vi "main.vi"() -> ()   [LabVIEW 2020]
uses:
  states_enum_typedef.ctl
  <vilib>/Analysis/baseanly.llb/Mean (DBL).vi
  <vilib>/addons/control/pid/pid.llb/PID (DBL).vi
  <vilib>/Analysis/NI_AALBase.lvlib
  <vilib>/addons/control/pid/NI_PID_pid.lvlib
panel:
  in  "Exit":bool
  in  "Tab Control":enum32{"Control", "Notes", "Profile", "Setup"}(tab)
  out "Zone 3\n Chart":dbl(graph)
  out "Zone 2 Chart":dbl(graph)
  out "Zone 1 Chart":dbl(graph)
  in  "Zone 1 SP":dbl
  in  "Zone 2 SP":dbl
  in  "Zone 3 SP":dbl
  out "Zone 1 Duty Cycle":dbl(knob) scale=0.0..100.0
  out "Zone 2 Duty Cycle":dbl(knob) scale=0.0..100.0
  out "Zone 3 Duty Cycle":dbl(knob) scale=0.0..100.0
  out "Z1":bool
  out "Z2":bool
  out "Z3":bool
  in  "Notes":string
  out "Profile Chart":dbl(graph)
  in  "Reset":bool
  out "Control Loop Stopped":bool
  out "Main Loop":i32
  out "PWM Loop":i32
  in  "Zone 1 PID":T1={"proportional gain (Kc)"=1.0, "integral time (Ti, min)"=0.01, "derivative time (Td, min)"=0.0} {"derivative time (Td, min)" format="%.3f"; "integral time (Ti, min)" format="%.3f"; "proportional gain (Kc)" format="%.3f"}
  in  "Zone 2 PID":T1={"proportional gain (Kc)"=1.0, "integral time (Ti, min)"=0.01, "derivative time (Td, min)"=0.0} {"derivative time (Td, min)" format="%.3f"; "integral time (Ti, min)" format="%.3f"; "proportional gain (Kc)" format="%.3f"}
  in  "Zone 3 PID":T1={"proportional gain (Kc)"=1.0, "integral time (Ti, min)"=0.01, "derivative time (Td, min)"=0.0} {"derivative time (Td, min)" format="%.3f"; "integral time (Ti, min)" format="%.3f"; "proportional gain (Kc)" format="%.3f"}
  out "Errors":errorcluster
  out "PWM Errors":errorcluster
  out "Zone 3":dbl(slide) scale=15.0..350.0
  out "Zone 2":dbl(slide) scale=15.0..350.0
  out "Zone 1":dbl(slide) scale=15.0..350.0
  # "Reflow Oven Controller"
  # "DegC"
  # "DegC"
  # "DegC"
  # "Any notes you type here will be saved and is a handy pad for future reference"
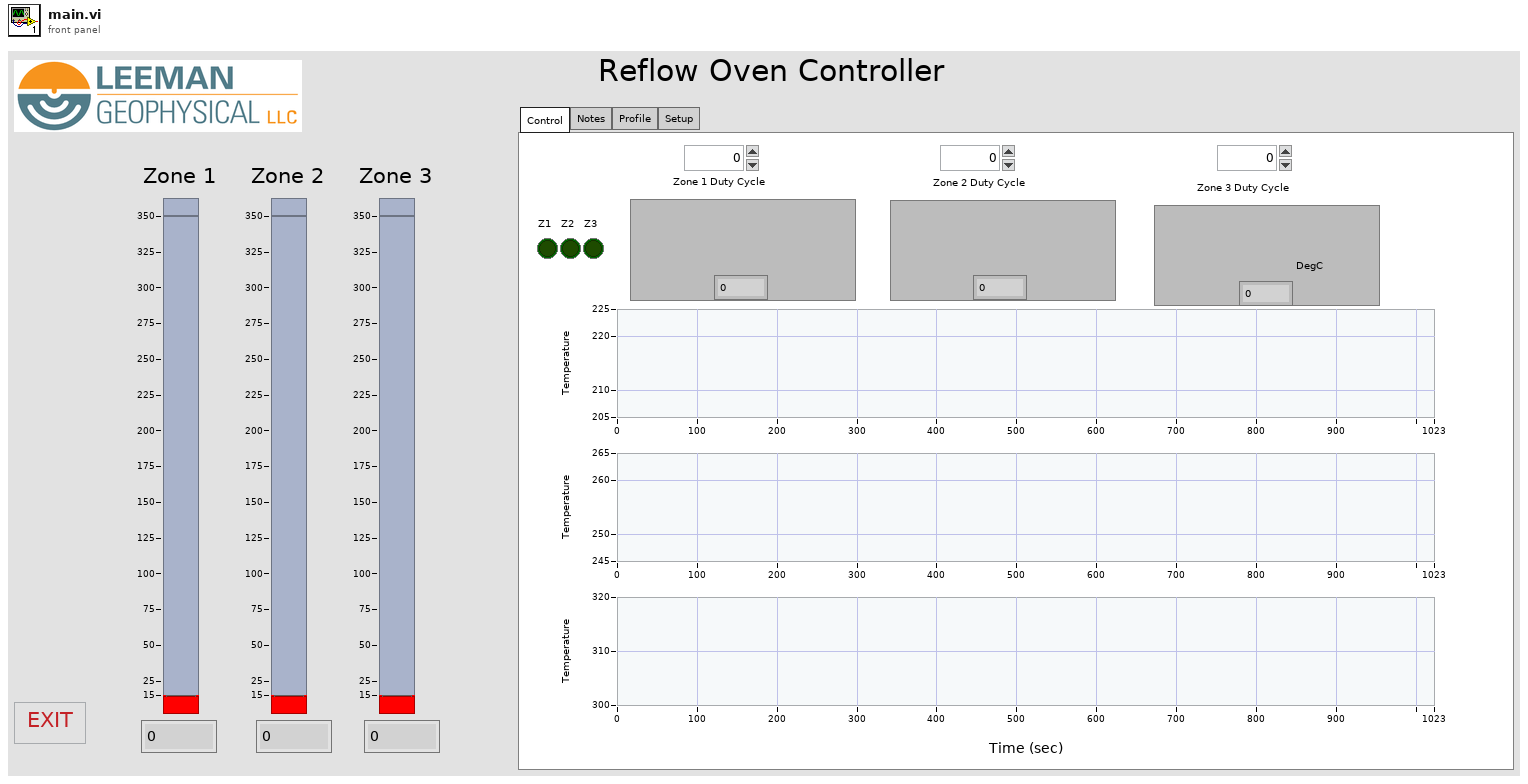
[diagram p1: front panel]
types:
  T1 = cluster{"proportional gain (Kc)":dbl, "integral time (Ti, min)":dbl, "derivative time (Td, min)":dbl}
  T2 = typedef "states_enum_typedef.ctl" = enum16{"Initilize", "Read", "Control 1", "Control 2", "Control 3", "Reset", "Wait", "Shutdown"}
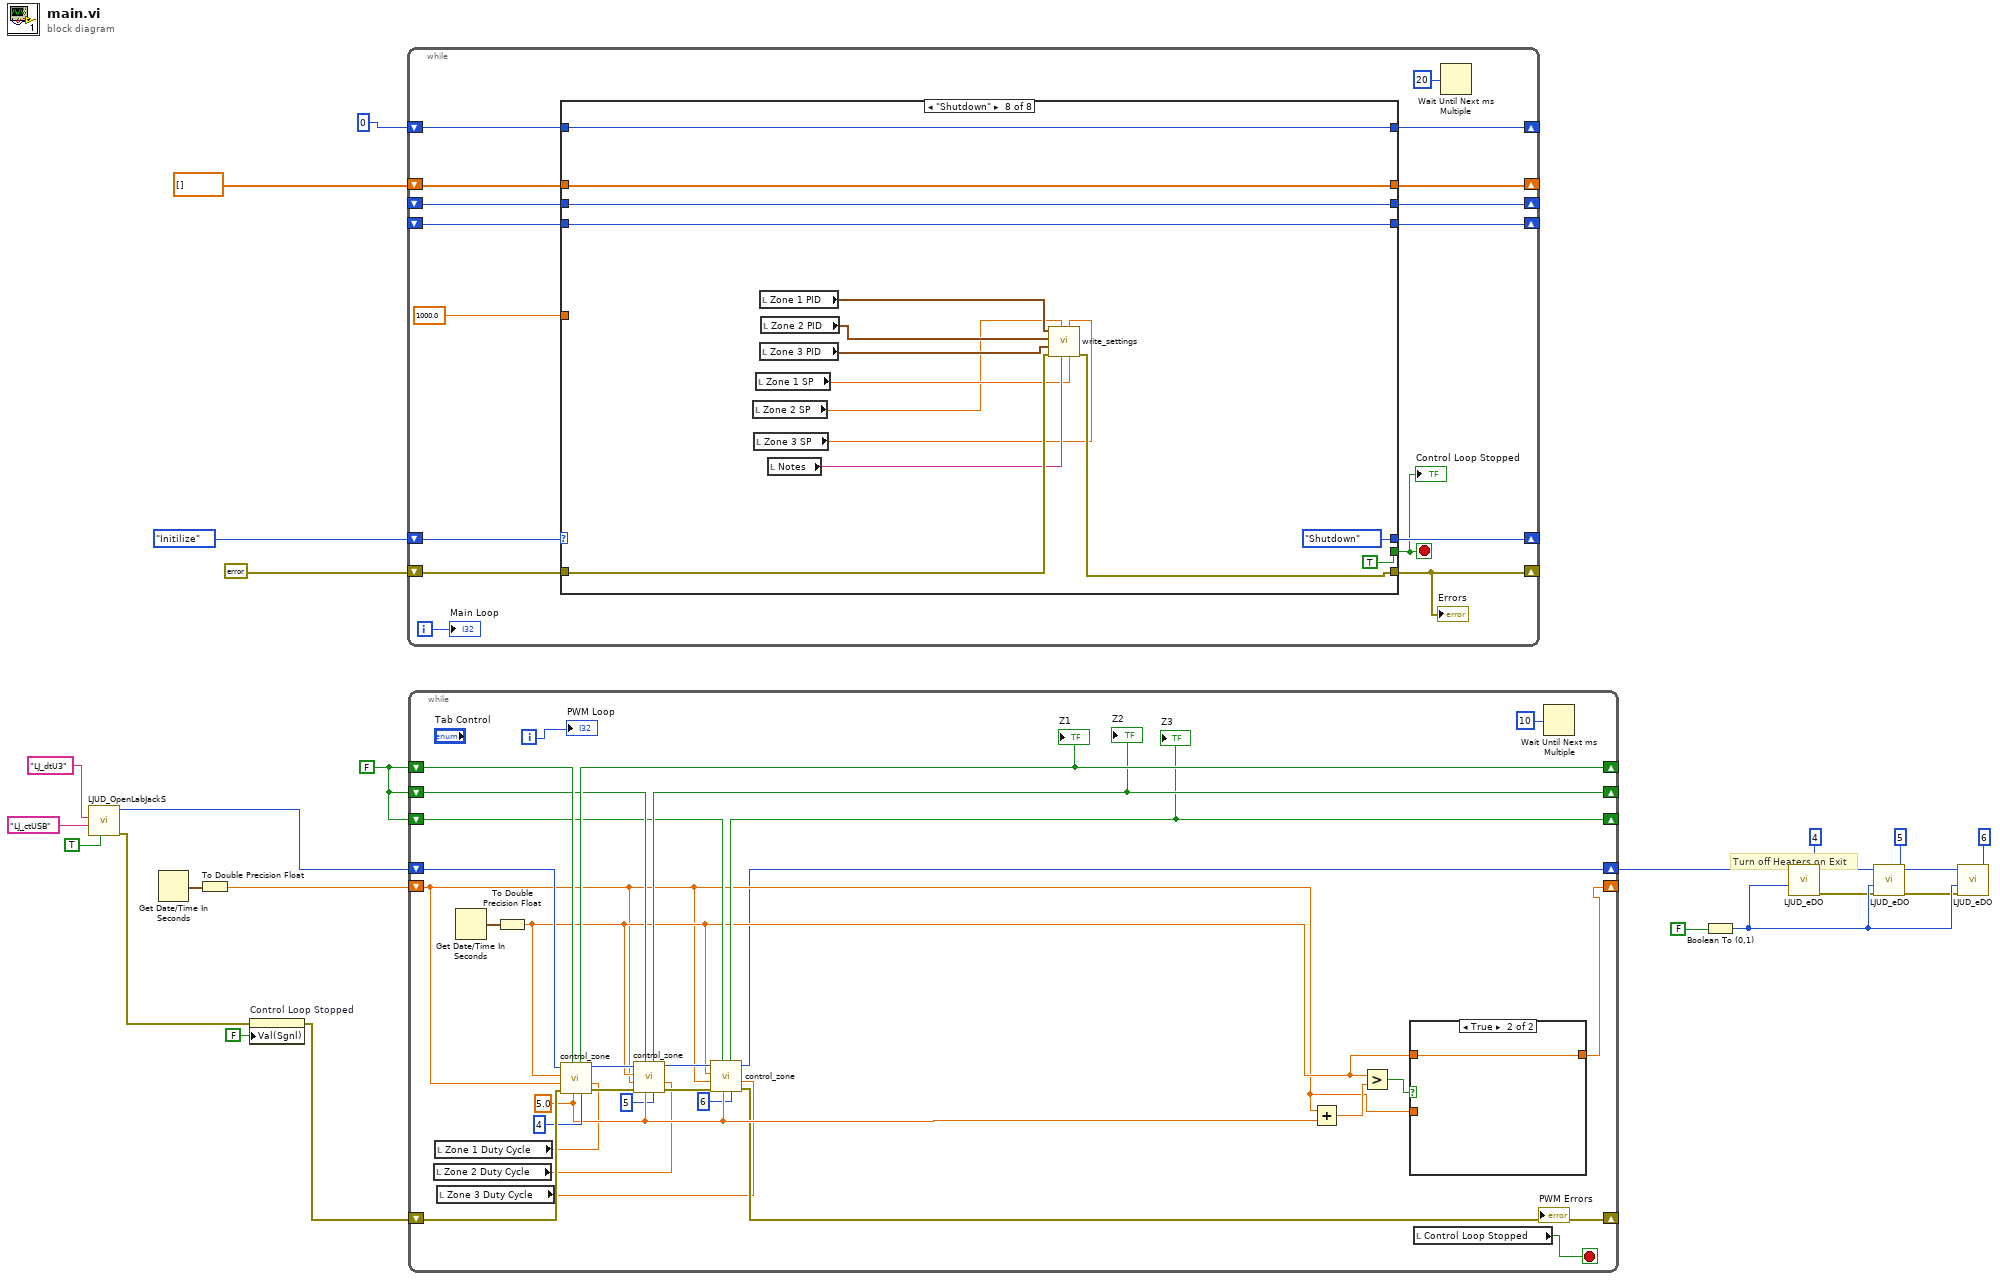
[diagram p0: block diagram]
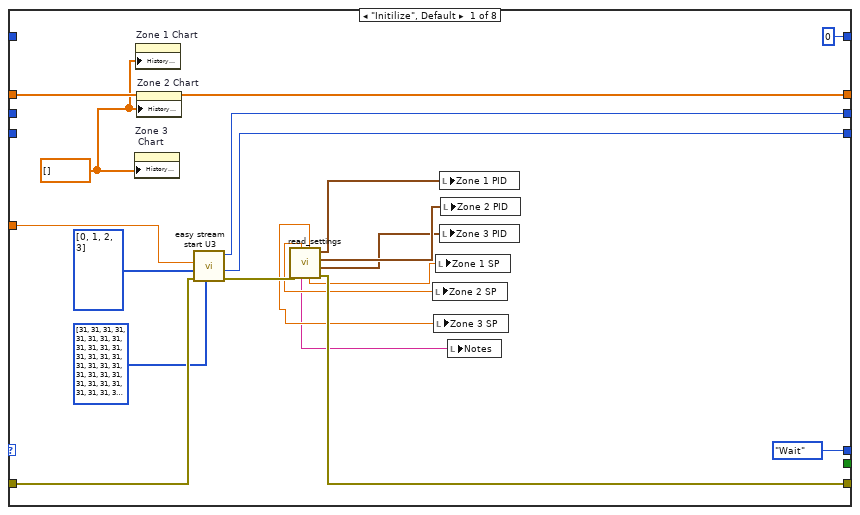
[diagram p3: hidden frame]
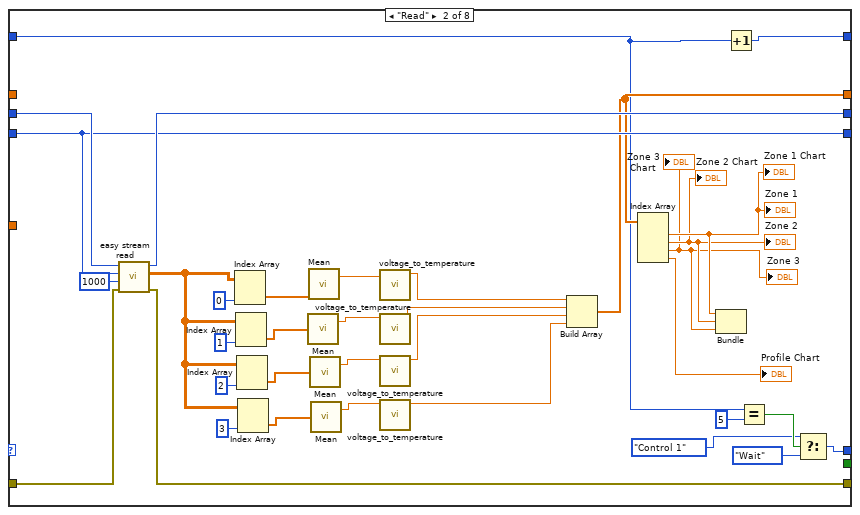
[diagram p4: hidden frame]
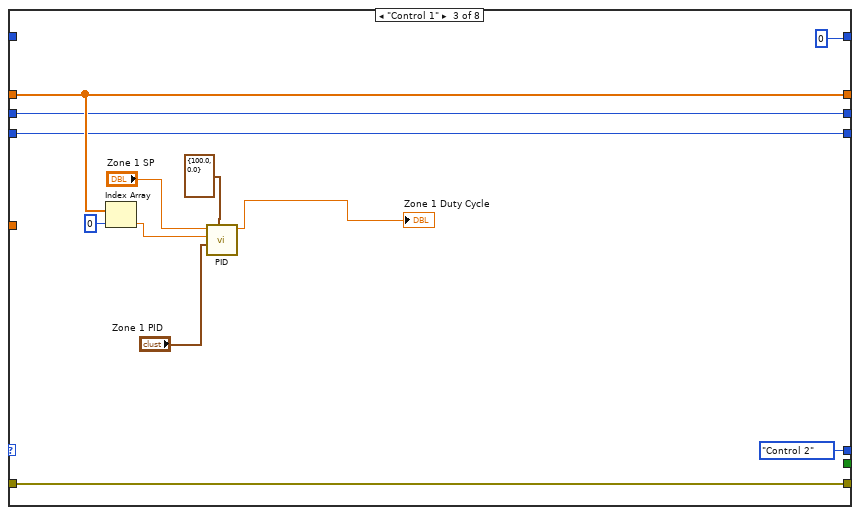
[diagram p5: hidden frame]
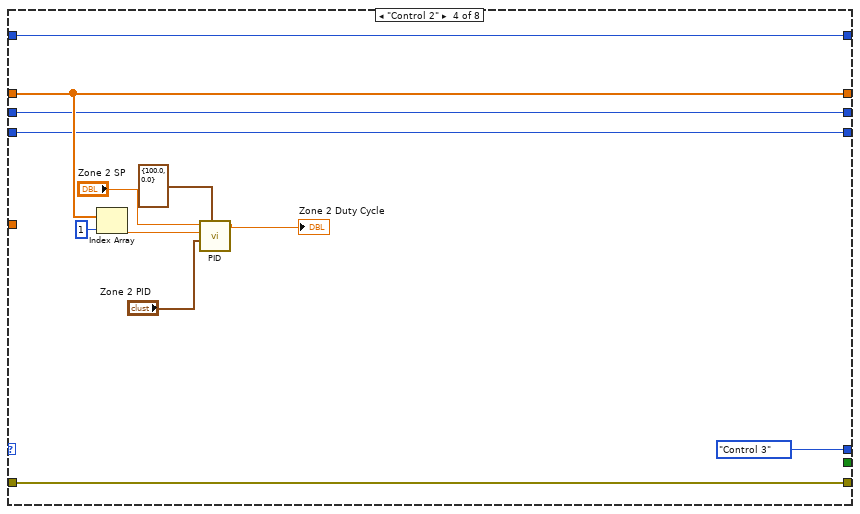
[diagram p6: hidden frame]
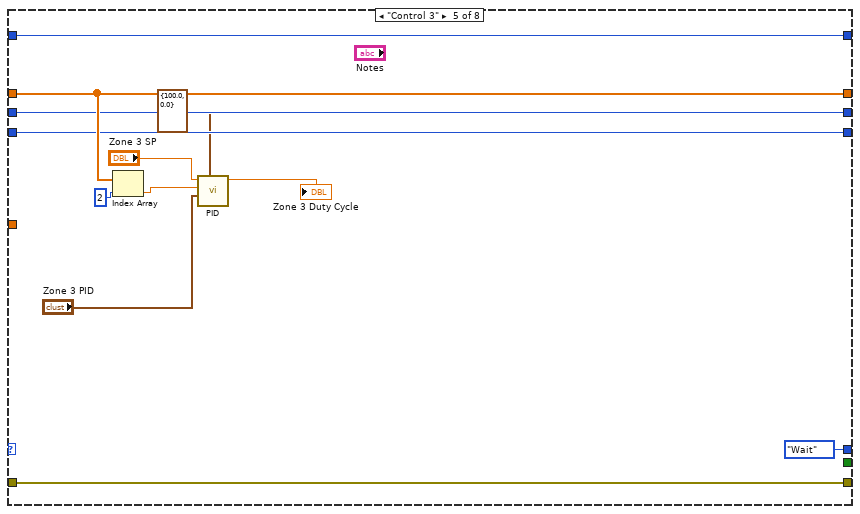
[diagram p7: hidden frame]
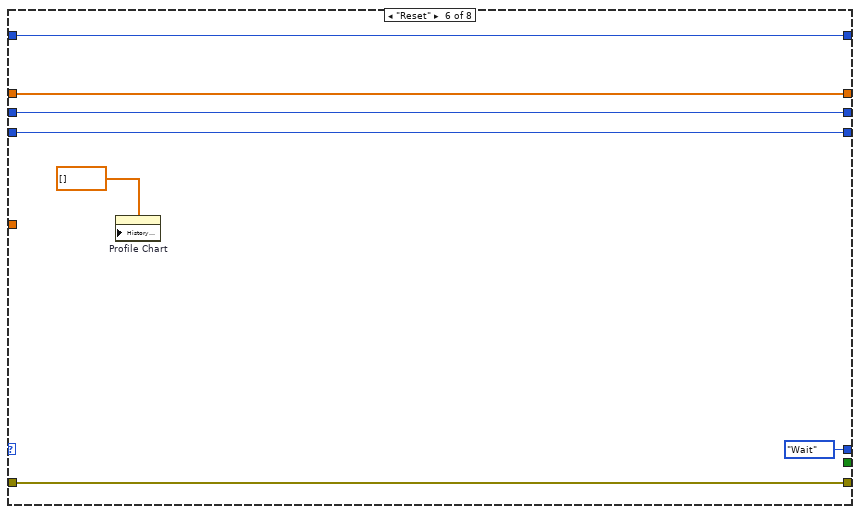
[diagram p8: hidden frame]
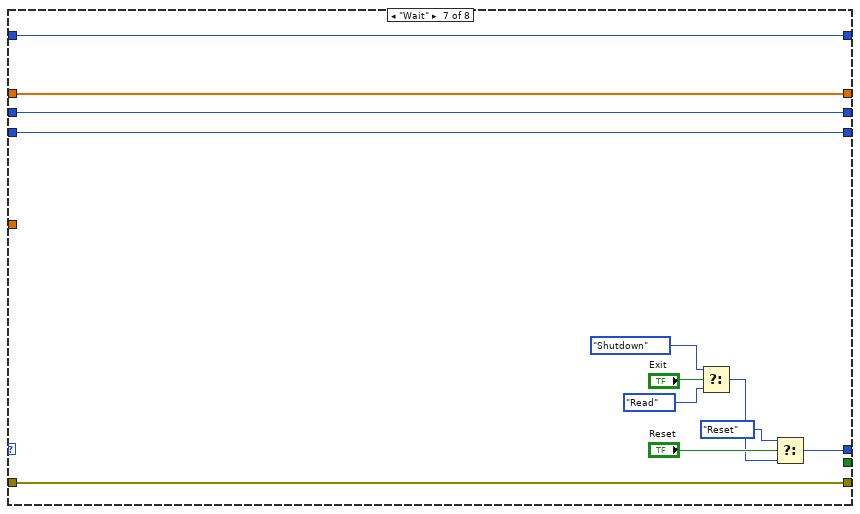
[diagram p9: hidden frame]
diagram:
  w2 = FALSE
  # "Turn off Heaters on Exit"
  n1 = call "LJUD_OpenLabJackS.vi"("FirstFound"=TRUE, "ConnectionType"="LJ_ctUSB", "DeviceType"="LJ_dtU3") -> ("error out"=w4:errorcluster, "Handle"=w6:i32)  [unwired: 6 in, 1 out]
  n2 = Get Date/Time In Seconds() -> (seconds since 1Jan1904=w8:timestamp)
  n3 = To Double Precision Float(number=w8) -> (double precision float=w7:dbl)
  n4 = property on="Control Loop Stopped" class="Bool (strict)"(error in=w4, "Val(Sgnl)"=FALSE ("Value (Signaling)")) -> (error out=w3:errorcluster)  [unwired: 1 in, 1 out]
  n5 = while {
    shift-right: [w39] -> _
    shift-left: states_enum_typedef."Initilize" -> [w30]
    shift-right: [w37] -> _
    shift-left: dbl[] [] -> [w40]
    shift-right: [w34] -> _
    shift-left: _ -> [w31]
    shift-right: [w35] -> _
    shift-left: _ -> [w32]
    shift-right: [w29] -> _
    shift-left: errorcluster {"status"=FALSE, "code"=0, "source"=""} ("error constant") -> [w36]
    shift-right: [w25] -> _
    shift-left: 0 -> [w26]
    i -> [w27]
    stop <- w28 stop-if-true
    n6 = case shown="\"Shutdown\"" w30 {
      tunnel: w40 -> [w58 _ w104 w118 w129 w136 w142 w162]
      tunnel: [states_enum_typedef."Wait" w62 states_enum_typedef."Control 2" states_enum_typedef."Control 3" states_enum_typedef."Wait" states_enum_typedef."Wait" w143 states_enum_typedef."Shutdown"] -> w39
      tunnel: [_ _ _ _ _ _ _ TRUE] -> w28
      tunnel: [w58 w79 w104 w118 w129 w136 w142 w162] -> w37
      tunnel: w36 -> [w56 w92 w101 w113 w125 w133 w139 w158]
      tunnel: [w55 w91 w103 w116 w127 w135 w141 w161] -> w35
      tunnel: [w54 w90 w102 w115 w126 w134 w140 w160] -> w34
      tunnel: 1000.0 ("Scan Rate (Hz)") -> [w53 _ _ _ _ _ _ _]
      tunnel: w32 -> [_ w94 w103 w116 w127 w135 w141 w161]
      tunnel: w31 -> [_ w90 w102 w115 w126 w134 w140 w160]
      tunnel: [w48 w89 w101 w113 w125 w133 w139 w157] -> w29
      tunnel: w26 -> [_ w60 _ w112 w124 w131 w138 w159]
      tunnel: [0 w61 0 w112 w124 w131 w138 w159] -> w25
      frame "Initilize", Default {
        w51 = dbl[] [] ("History Data")
        n7 = property on="Zone 3\n Chart" class="WFChart (strict)"("History Data"=w51) -> ()  [unwired: 2 in, 2 out]
        n8 = property on="Zone 1 Chart" class="WFChart (strict)"("History Data"=w51) -> ()  [unwired: 2 in, 2 out]
        n9 = property on="Zone 2 Chart" class="WFChart (strict)"("History Data"=w51) -> ()  [unwired: 2 in, 2 out]
        n10 = call "easy stream start U3.vi"("Scan List (-)"=u8[] [31, 31, 31, 31, 31, 31, 31, 31, 31, 31, 31, 31, 31, 31, 31, 31, 31, 31, 31, 31, 31, 31, 31, 31, 31, 31, 31, 31, 31, 31, 31, 31, 31, 31, 31, 31, 31, 31, 31, 31, 31, 31, 31, 31, 31, 31, 31, 31, 31, 31, 31, 31, 31, 31, 31, 31, 31, 31, 31, 31, 31, 31, 31, 31, 31, 31, 31, 31, 31, 31, 31, 31, 31, 31, 31, 31, 31, 31, 31, 31, 31, 31, 31, 31, 31, 31, 31, 31, 31, 31, 31, 31, 31, 31, 31, 31, 31, 31, 31, 31, 31, 31, 31, 31, 31, 31, 31, 31, 31, 31, 31, 31, 31, 31, 31, 31, 31, 31, 31, 31, 31, 31, 31, 31, 31, 31, 31, 31], "error in"=w56, "Scan List (+)"=u8[] [0, 1, 2, 3], "Scan Rate (Hz)"=w53) -> ("error out"=w49:errorcluster, "# Channels"=w54:i32, "Handle Out"=w55:i32)  [unwired: 4 in, 1 out]
        n11 = call "read_settings.vi"("error in"=w49) -> ("error out"=w48:errorcluster, "Zone 3 PID"=w45:T1, "Zone 2 PID"=w46:T1, "Zone 1 PID"=w47:T1, "Zone 1 SP"=w44:dbl, "Zone 3 SP"=w42:dbl, "Notes"=w41:string, "Zone 2 SP"=w43:dbl)  [unwired: 3 in]
        n12 = local write "Zone 2 SP"(w43) -> ()
        n13 = local write "Zone 3 SP"(w42) -> ()
        n14 = local write "Zone 1 SP"(w44) -> ()
        n15 = local write "Zone 1 PID"(w47) -> ()
        n16 = local write "Zone 3 PID"(w45) -> ()
        n17 = local write "Zone 2 PID"(w46) -> ()
        n18 = local write "Notes"(w41) -> ()
      }
      frame "Read" {
        n19 = call "easy stream read.vi"("error in"=w92, "Scans To Read"=1000, "# Channels In Stream"=w90, "Handle In"=w94) -> ("error out"=w89:errorcluster, "Data"=w84:dbl[][], "Handle Out"=w91:i32)  [unwired: 4 in, 1 out]
        n20 = Index Array(array=w84, index (col)=0 ("disabled index (col)")) -> (element=w83:dbl[])  [unwired: 1 in]
        n21 = Index Array(array=w84, index (col)=1 ("disabled index (col)")) -> (element=w82:dbl[])  [unwired: 1 in]
        n22 = Index Array(array=w84, index (col)=2 ("disabled index (col)")) -> (element=w81:dbl[])  [unwired: 1 in]
        n23 = Index Array(array=w84, index (col)=3 ("disabled index (col)")) -> (element=w80:dbl[])  [unwired: 1 in]
        n24 = call-poly <vilib>:"Mean.vi"("X"=w82) -> ("mean"=w77:dbl)  [unwired: 1 out]
        n25 = call-poly <vilib>:"Mean.vi"("X"=w83) -> ("mean"=w78:dbl)  [unwired: 1 out]
        n26 = call-poly <vilib>:"Mean.vi"("X"=w81) -> ("mean"=w76:dbl)  [unwired: 1 out]
        n27 = call-poly <vilib>:"Mean.vi"("X"=w80) -> ("mean"=w75:dbl)  [unwired: 1 out]
        n28 = call "voltage_to_temperature.vi"("Voltage In"=w78) -> ("Temp Out"=w72:dbl)  [unwired: 9 in, 1 out]
        n29 = call "voltage_to_temperature.vi"("Voltage In"=w77) -> ("Temp Out"=w71:dbl)  [unwired: 9 in, 1 out]
        n30 = call "voltage_to_temperature.vi"("Voltage In"=w76) -> ("Temp Out"=w73:dbl)  [unwired: 9 in, 1 out]
        n31 = call "voltage_to_temperature.vi"("Voltage In"=w75) -> ("Temp Out"=w74:dbl)  [unwired: 9 in, 1 out]
        n32 = Build Array(w72, w71, w73, w74) -> (w79:dbl[])
        n33 = Index Array(array=w79) -> (element #1=w69:dbl, element #2=w68:dbl, element #3=w67:dbl, element #4=→"Profile Chart":dbl)  [unwired: 4 in]
        "Zone 1" <- w69
        "Zone 2" <- w68
        "Zone 3" <- w67
        "Zone 1 Chart" <- w69
        "Zone 2 Chart" <- w68
        "Zone 3\n Chart" <- w67
        n34 = Bundle("Temp Out"=w69, "Temp Out"=w68, "Temp Out"=w67) -> ()  [unwired: 1 in, 1 out]
        n35 = Increment(x=w60) -> (x+1=w61:i32)
        n36 = Equal?(x=w60, y=5) -> (x = y?=w65:bool)
        n37 = Select(t=states_enum_typedef."Control 1", s=w65, f=states_enum_typedef."Wait") -> (s? t:f=w62:T2)
      }
      frame "Control 1" {
        n38 = Index Array(array=w104, index=0) -> (element=w97:dbl)
        n39 = call-poly <vilib>:"PID.vi"("output range"=cluster{"output high":dbl, "output low":dbl} {"output high"=100.0, "output low"=0.0}, "PID gains"="Zone 1 PID", "process variable"=w97, "setpoint"="Zone 1 SP") -> ("output"=→"Zone 1 Duty Cycle":dbl)  [unwired: 6 in, 1 out]
      }
      frame "Control 2" {
        n40 = Index Array(array=w118, index=1) -> (element=w109:dbl)
        n41 = call-poly <vilib>:"PID.vi"("output range"=cluster{"output high":dbl, "output low":dbl} {"output high"=100.0, "output low"=0.0}, "PID gains"="Zone 2 PID", "process variable"=w109, "setpoint"="Zone 2 SP") -> ("output"=→"Zone 2 Duty Cycle":dbl)  [unwired: 6 in, 1 out]
      }
      frame "Control 3" {
        n42 = Index Array(array=w129, index=2) -> (element=w121:dbl)
        n43 = call-poly <vilib>:"PID.vi"("output range"=cluster{"output high":dbl, "output low":dbl} {"output high"=100.0, "output low"=0.0}, "PID gains"="Zone 3 PID", "process variable"=w121, "setpoint"="Zone 3 SP") -> ("output"=→"Zone 3 Duty Cycle":dbl)  [unwired: 6 in, 1 out]
      }
      frame "Reset" {
        n44 = property on="Profile Chart" class="WFChart (strict)"("History Data"=dbl[] []) -> ()  [unwired: 2 in, 2 out]
      }
      frame "Wait" {
        n45 = Select(t=states_enum_typedef."Shutdown", s="Exit", f=states_enum_typedef."Read") -> (s? t:f=w147:T2)
        n46 = Select(t=states_enum_typedef."Reset", s="Reset", f=w147) -> (s? t:f=w143:T2)
      }
      frame "Shutdown" {
        n47 = local read "Zone 2 SP"() -> (w151:dbl)
        n48 = local read "Zone 3 SP"() -> (w150:dbl)
        n49 = local read "Zone 1 SP"() -> (w155:dbl)
        n50 = local read "Zone 1 PID"() -> (w154:T1)
        n51 = local read "Zone 3 PID"() -> (w152:T1)
        n52 = local read "Zone 2 PID"() -> (w153:T1)
        n53 = local read "Notes"() -> (w156:string)
        n54 = call "write_settings.vi"("Zone 1 SP"=w155, "Zone 3 SP"=w150, "Notes"=w156, "Zone 2 SP"=w151, "error in"=w158, "Zone 3 PID"=w152, "Zone 2 PID"=w153, "Zone 1 PID"=w154) -> ("error out"=w157:errorcluster)  [unwired: 3 in]
      }
    }
    "Errors" <- w29
    "Control Loop Stopped" <- w28
    n55 = Wait Until Next ms Multiple(millisecond multiple=u32 20) -> ()  [unwired: 1 out]
    "Main Loop" <- w27
  }
  n56 = while {
    shift-right: [w189] -> _
    shift-left: w7 -> [w170]
    shift-right: [w183] -> _
    shift-left: w2 -> [w184]
    shift-right: [w169] -> w5
    shift-left: w6 -> [w187]
    shift-right: [w168] -> _
    shift-left: w3 -> [w186]
    shift-right: [w174] -> _
    shift-left: w2 -> [w175]
    shift-right: [w172] -> _
    shift-left: w2 -> [w173]
    i -> [w192]
    stop <- w193 stop-if-true
    w180 = 5.0 ("total cycle time")
    n57 = local read "Zone 2 Duty Cycle"() -> (w166:dbl)
    n58 = local read "Zone 1 Duty Cycle"() -> (w167:dbl)
    n59 = local read "Zone 3 Duty Cycle"() -> (w165:dbl)
    n60 = Get Date/Time In Seconds() -> (seconds since 1Jan1904=w194:timestamp)
    n61 = To Double Precision Float(number=w194) -> (double precision float=w171:dbl)
    n62 = call "control_zone.vi"("duty cycle in"=w167, "Channel"=4, "total cycle time"=w180, "Last State"=w184, "error in"=w186, "Seq Start Time"=w170, "Now Time"=w171, "Handle In"=w187) -> ("error out"=w182:errorcluster, "Handle Out"=w176:i32, "state out"=w183:bool)  [unwired: 1 in]
    "Z1" <- w183
    n63 = call "control_zone.vi"("duty cycle in"=w166, "Channel"=5, "total cycle time"=w180, "Last State"=w175, "error in"=w182, "Seq Start Time"=w170, "Now Time"=w171, "Handle In"=w176) -> ("error out"=w181:errorcluster, "Handle Out"=w177:i32, "state out"=w174:bool)  [unwired: 1 in]
    "Z2" <- w174
    n64 = call "control_zone.vi"("duty cycle in"=w165, "Channel"=6, "total cycle time"=w180, "Last State"=w173, "error in"=w181, "Seq Start Time"=w170, "Now Time"=w171, "Handle In"=w177) -> ("error out"=w168:errorcluster, "Handle Out"=w169:i32, "state out"=w172:bool)  [unwired: 1 in]
    "PWM Errors" <- w168
    "Z3" <- w172
    n65 = Add(x=w170, y=w180) -> (x+y=w191:dbl)
    n66 = Greater?(x=w171, y=w191) -> (0:w190:bool)
    n67 = case shown="True" w190 {
      tunnel: [w195 w196] -> w189
      tunnel: w171 -> [_ w196]
      tunnel: w170 -> [w195 _]
      frame False {
      }
      frame True {
      }
    }
    n68 = local read "Control Loop Stopped"() -> (w193:bool)
    n69 = Wait Until Next ms Multiple(millisecond multiple=u32 10) -> ()  [unwired: 1 out]
    "PWM Loop" <- w192
  }
  n70 = Boolean To (0,1)(Boolean=FALSE) -> (0, 1=w16:i16)
  n71 = call "LJUD_eDO.vi"("State"=w16, "Channel"=4, "Handle In"=w5) -> ("error out"=w14:errorcluster, "Handle Out"=w17:i32)  [unwired: 7 in]
  n72 = call "LJUD_eDO.vi"("error in"=w14, "State"=w16, "Channel"=5, "Handle In"=w17) -> ("error out"=w15:errorcluster, "Handle Out"=w18:i32)  [unwired: 6 in]
  n73 = call "LJUD_eDO.vi"("error in"=w15, "State"=w16, "Channel"=6, "Handle In"=w18) -> ()  [unwired: 6 in, 2 out]
